vi "SLM Control.vi"(7 "Calling VI Ref":refnum<vi>) -> ()   [LabVIEW 2018]
uses:
  SLM Control TypeDefs/SLM Ctrl Mode Names.ctl
  <vilib>/Utility/miscctls.llb/LVPointTypeDef.ctl
  Device Library/Spatial Light Modulator/SLM Polymorphic Messenger/Get Status.vi
  Device Library/Spatial Light Modulator/SLM Polymorphic Messenger/Set Flat File.vi
  Device Library/Spatial Light Modulator/SLM Polymorphic Messenger/Number of Modes.vi
  Device Library/Spatial Light Modulator/SLM Polymorphic Messenger/Holo Size.vi
  Device Library/Spatial Light Modulator/SLM Polymorphic Messenger/Flat On or Off.vi
  Device Library/Spatial Light Modulator/SLM Polymorphic Messenger/Vortex On or Off.vi
  Device Library/Spatial Light Modulator/SLM Polymorphic Messenger/Toggle Vortex Direction.vi
  Device Library/Spatial Light Modulator/SLM Polymorphic Messenger/Top Hat On or Off.vi
  Device Library/Spatial Light Modulator/SLM Polymorphic Messenger/Top Hat Size.vi
  Device Library/Spatial Light Modulator/SLM Polymorphic Messenger/Mode Amplitude.vi
  Device Library/Spatial Light Modulator/SLM Polymorphic Messenger/Holo Position.vi
panel:
  out "Flat File":string
  in  "Center Holo":bool
  in  "X Pos Minus":bool
  in  "X Pos Plus":bool
  in  "Y Pos Minus":bool
  in  "Y Pos Plus":bool
  in  "Hologram Y Position":i32=20 min=1 max=1000
  in  "Hologram X Position":i32=20 min=1 max=1000
  in  "Set Flat File":bool
  in  "Clear All":bool
  in  "Set Zero":bool
  in  "Quit":bool
  in  "Notifier Name":string
  out "SLM Image":T1(plugin-control)
  in  "Active SLM":u16(ring) items=["Test"]
  in  "Hologram Diameter (px)":i32=20
  in  "Top Hat Radius":dbl=20.0
  in  "SLM Flat":bool
  in  "Vortex Direction":bool
  in  "Top Hap":bool
  in  "Mode Step Plus":bool
  in  "Mode Step Minus":bool
  in  "Current Mode":i32(ring) items=["Tip", "Tilt", "Defocus", "Astigmatism 90", "Astigmatism 45", "Coma 01", "Coma 02", "Trefoil 01", "Trefoil 02", "1st Spherical", "12", "13", "14", "15", "16", "17", "18", "19"]
  in  "Mode Amount":dbl
  in  "Step Size":dbl
  in  "Amp Step Plus":bool
  in  "Amp Step Minus":bool
  out "Error":bool
  in  "Number of Modes":i32=20 min=0 max=32
  in  "Vortex":bool
  out "Mode Plot":cluster{dbl[], dbl[]}(graph)
  # "SLM Display"
  # "Current Mode"
  # "Amplitude"
  # "Increment"
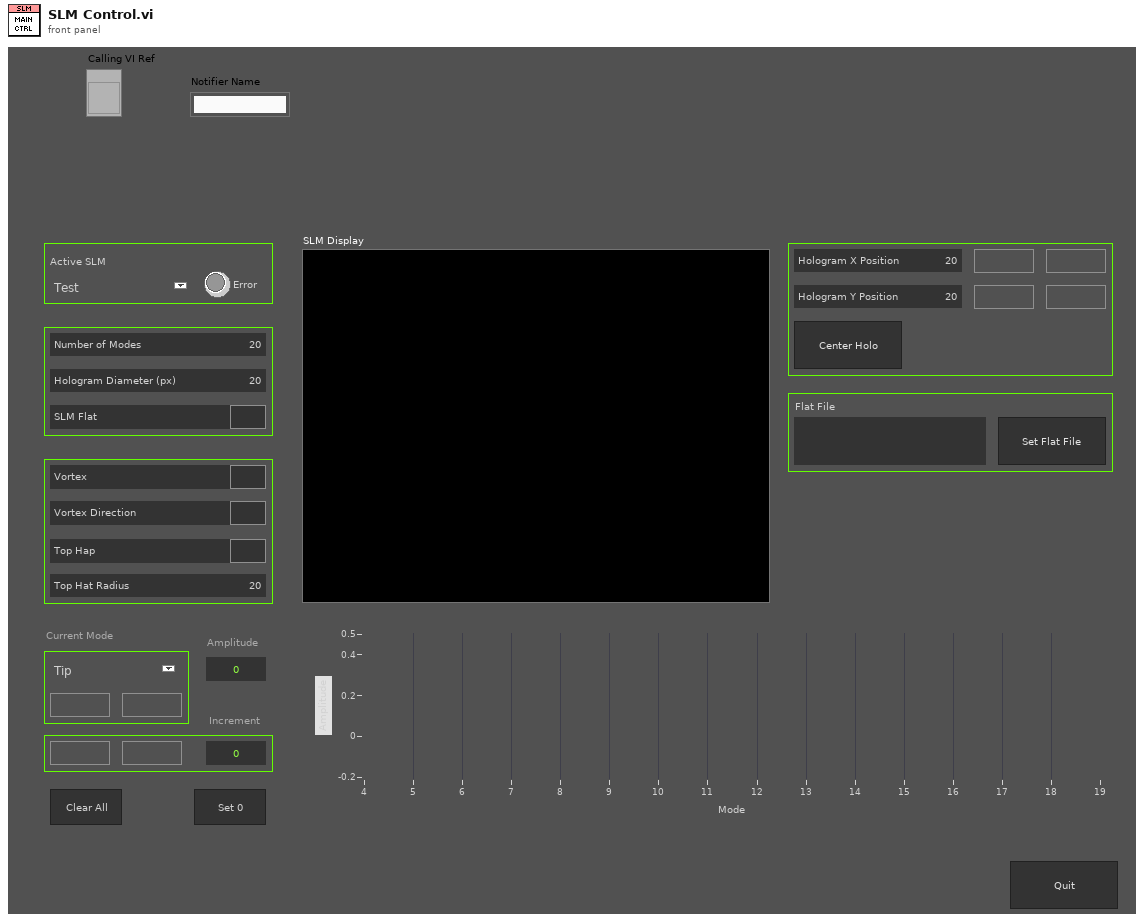
[diagram p1: front panel]
types:
  T1 = typedef "IMAQ Image.ctl" = refnum<image>
  T2 = enum16{"Always On", "Always Off", "Off While Running"}
  T3 = typedef "LVPointTypeDef.ctl" = cluster{"Horizontal":i16, "Vertical":i16}
  T4 = typedef "SLM Ctrl Mode Names.ctl" = cluster{"ModeNumbers":i32[], "ModeNames":string[]}
  T5 = typedef "X10468 SLM Notifier.ctl" = cluster{"SLM Actions":T6, "SLM Image":T1, "Flat On?":bool, "Vortex On?":bool, "Top Hat On?":bool, "Mode Amps":dbl[], "Number of Modes":i32, "Holo Diameter (px)":i32, "Top Hat Radius":dbl, "Holo Position":i32[], "Received?":bool, "Flat File Path":path}
  T6 = typedef "X10468 SLM Actions.ctl" = enum16{"Exit Loop", "Get Settings", "Set Flat File", "Change Holo Size", "Change Num Modes", "Change Holo Position", "Change Top Hat Size", "Change Vortex Direction", "Change Mode Amounts", "Flat On/Off", "Vortex On/Off", "Top Hat On/Off", "Make Hologram", "Update SLM Display", "Quit"}
  T7 = typedef "LVRectTypeDef.ctl" = cluster{"Left":i16, "Top":i16, "Right":i16, "Bottom":i16}
  T8 = typedef "LVBoundsTypeDef.ctl" = cluster{"Width":u32, "Height":u32}
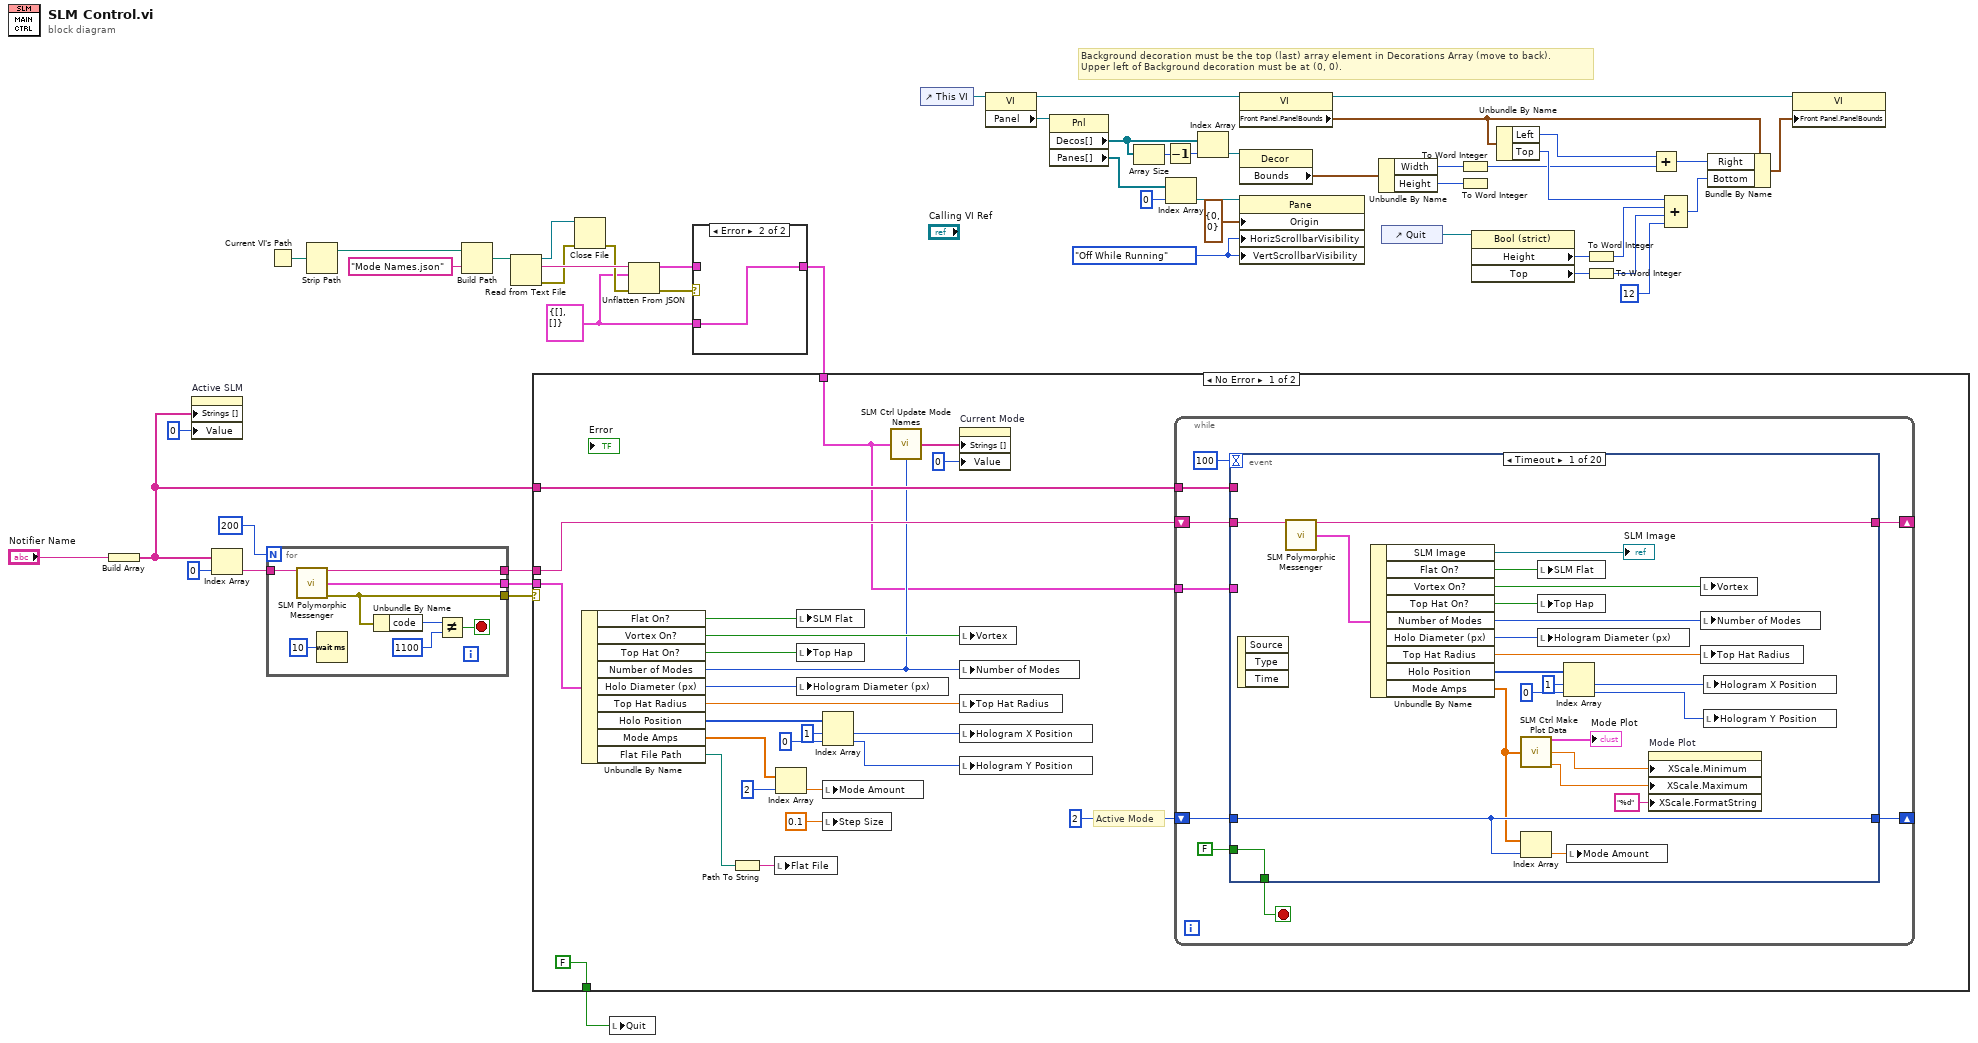
[diagram p0: block diagram]
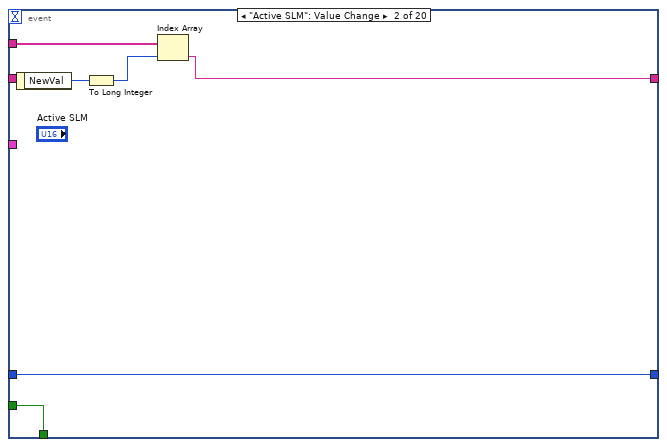
[diagram p2: hidden frame]
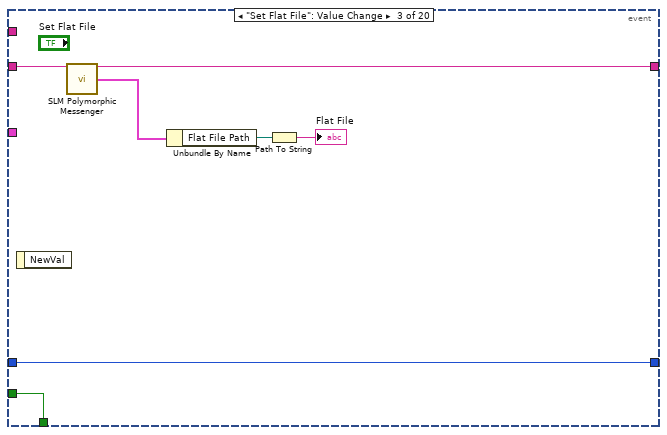
[diagram p3: hidden frame]
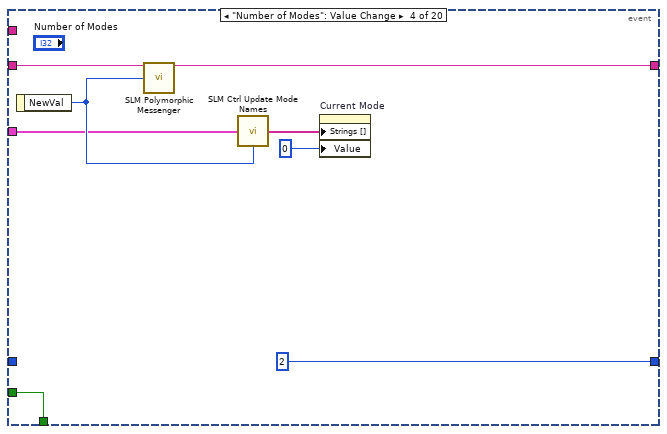
[diagram p4: hidden frame]
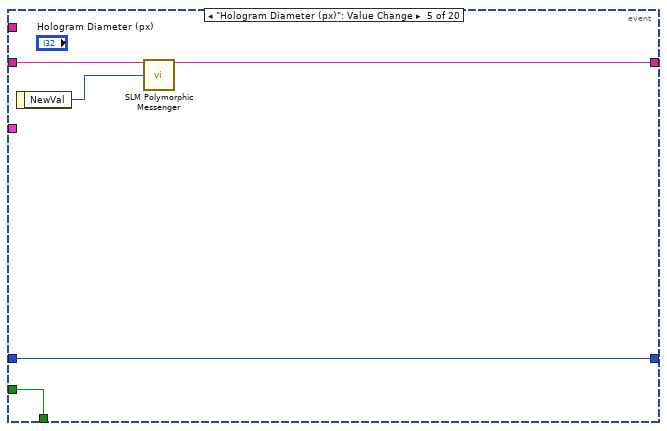
[diagram p5: hidden frame]
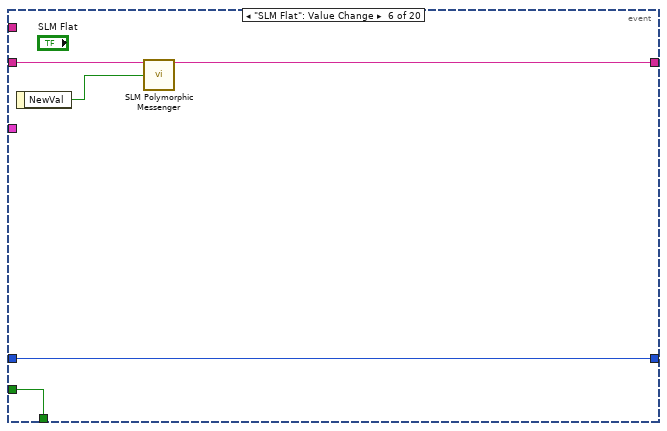
[diagram p6: hidden frame]
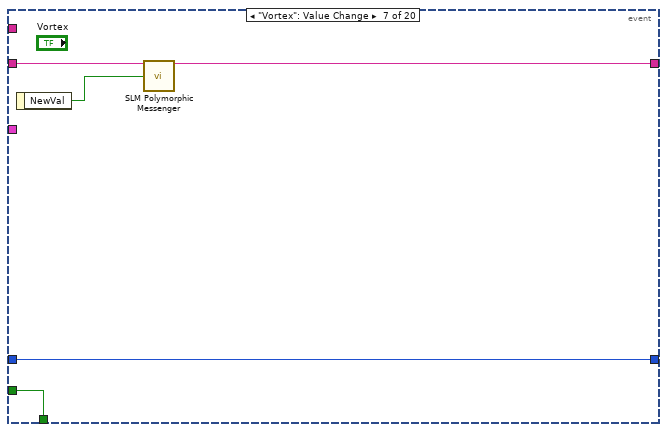
[diagram p7: hidden frame]
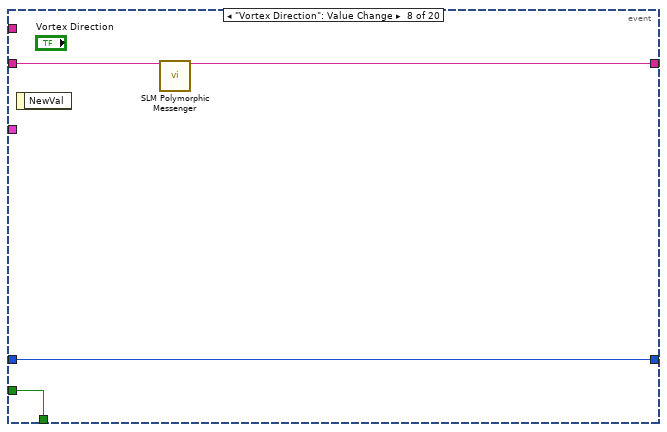
[diagram p8: hidden frame]
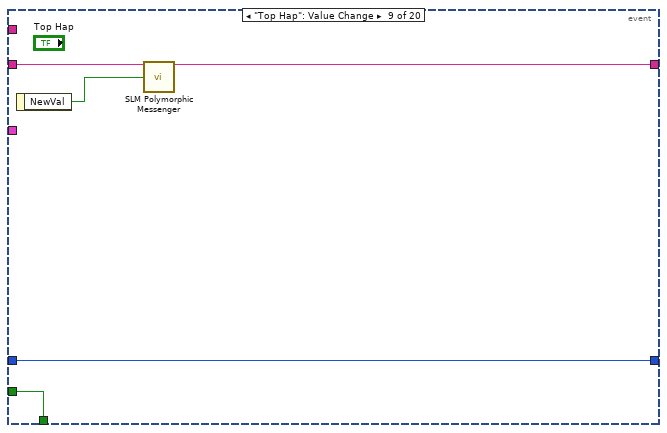
[diagram p9: hidden frame]
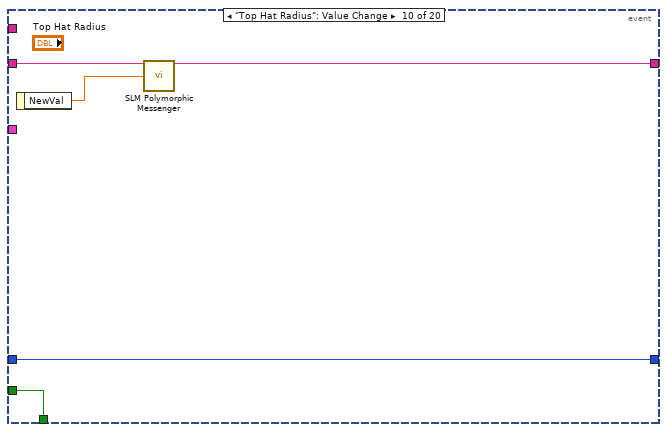
[diagram p10: hidden frame]
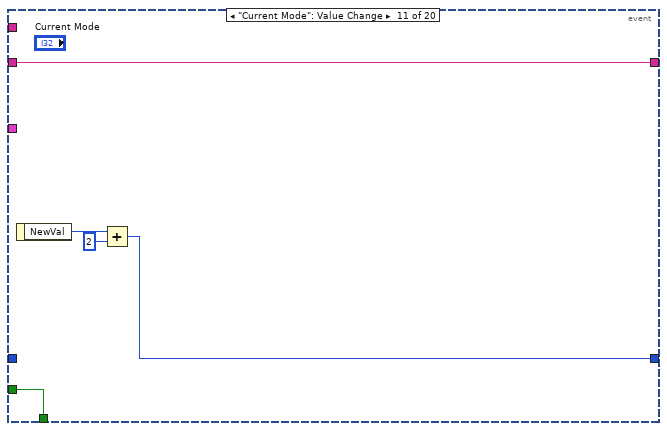
[diagram p11: hidden frame]
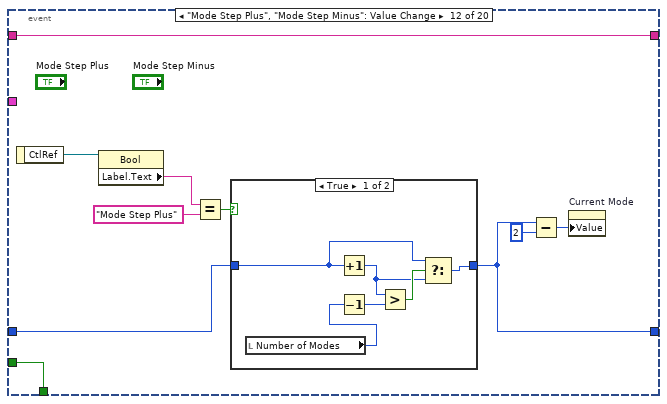
[diagram p12: hidden frame]
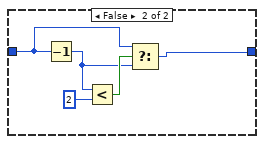
[diagram p13: hidden frame]
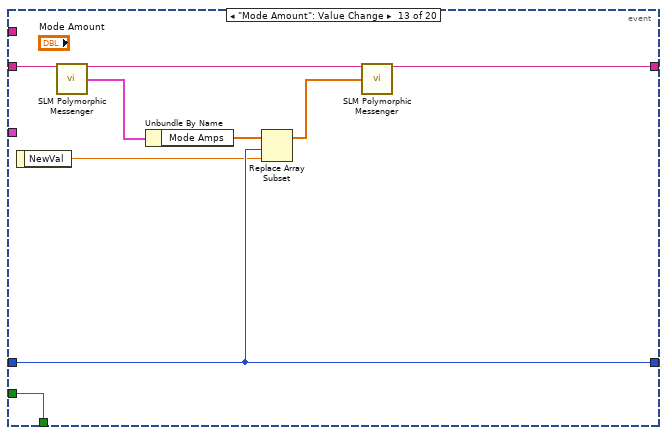
[diagram p14: hidden frame]
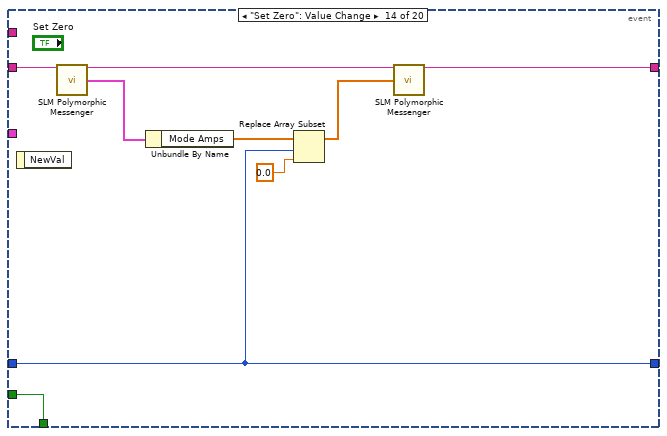
[diagram p15: hidden frame]
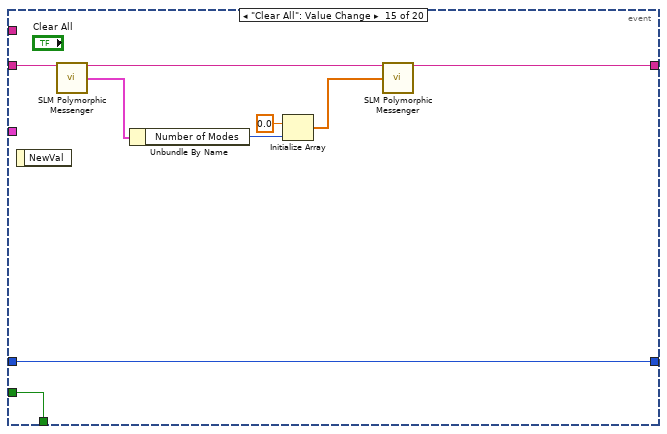
[diagram p16: hidden frame]
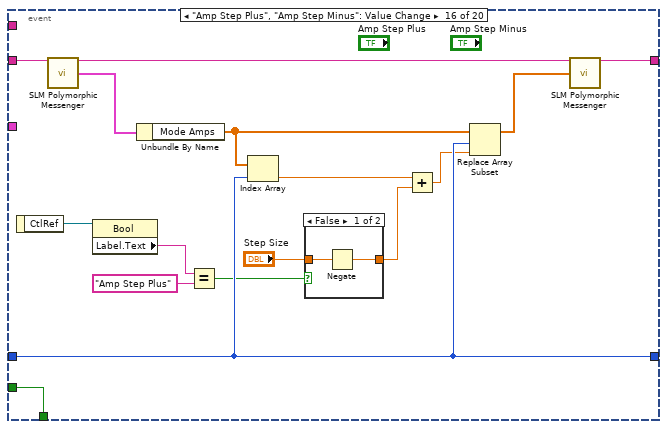
[diagram p17: hidden frame]
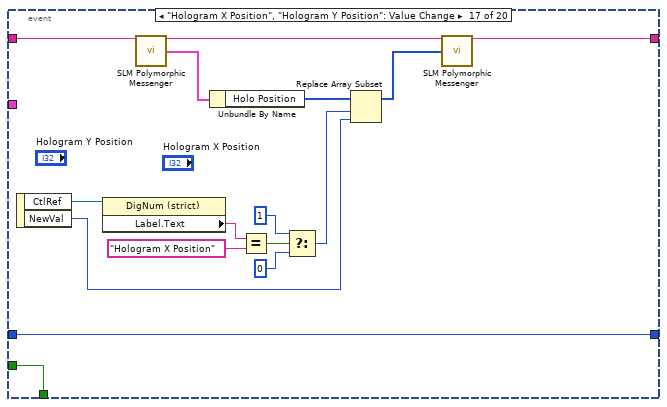
[diagram p19: hidden frame]
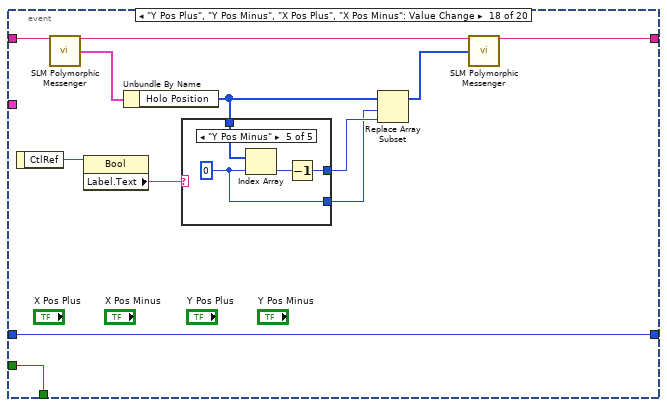
[diagram p20: hidden frame]
diagram:
  w12 = T2."Off While Running" ("Vertical Scrollbar Visibility")
  w37 = T4 {"ModeNumbers"=[], "ModeNames"=[]} ("ModeNamesArray")
  # "Background decoration must be the top (last) array element in Decorations Array (move to back).\nUpper left of Background decoration must be at (0, 0)."
  n1 = Build Array("Notifier Name") -> (w48:string[])
  n2 = property on="Active SLM" class="Ring (strict)"("Strings []"=w48, "Value"=u16 0) -> ()  [unwired: 2 in, 2 out]
  n3 = Index Array(array=w48, index=0) -> (element=w35:string)
  n4 = for {
    N: 200 -> [_]
    tunnel: [w56] -> w34
    tunnel: w35 -> [w54]
    tunnel: [w53] -> w33
    tunnel: [w52] -> w32
    stop <- w57 stop-if-true
    n5 = call-poly "SLM Polymorphic Messenger.vi"("Notifier Name"=w54) -> ("Notifier Name Dup"=w53:string, "SLM Status"=w52:T5, "Error Out"=w56:errorcluster)  [unwired: 12 in]
    n6 = Wait (ms)(milliseconds to wait=u32 10) -> ()  [unwired: 1 out]
    n7 = Unbundle By Name(w56) -> ("code"=w59:i32)
    n8 = Not Equal?(x=w59, y=1100 ("x")) -> (x != y?=w57:bool)
  }
  n9 = Current VI's Path() -> (path=w47:path)
  n10 = Strip Path(path=w47) -> (stripped path=w46:path)  [unwired: 1 out]
  n11 = Build Path(base path=w46, name or relative path="Mode Names.json") -> (appended path=w44:path)
  n12 = Read from Text File(file (use dialog)=w44) -> (refnum out=w42:refnum<file>, text=w43:string, error out=w41:errorcluster)  [unwired: 3 in, 1 out]
  n13 = Close File(refnum=w42, error in=w41) -> (error out=w40:errorcluster)  [unwired: 1 out]
  n14 = Unflatten From JSON(JSON string=w43, type and defaults=w37, error in (no error)=w40) -> (value=w38:T4, error out=w39:errorcluster)  [unwired: 4 in]
  n15 = case shown="Error" w39 {
    tunnel: w38 -> [w60 _]
    tunnel: [w60 w61] -> w31
    tunnel: w37 -> [_ w61]
    frame No Error {
    }
    frame Error {
    }
  }
  n16 = case shown="No Error" w34 {
    tunnel: w48 -> [w86 _]
    tunnel: w33 -> [w84 _]
    tunnel: w32 -> [w85 _]
    tunnel: w31 -> [w68 _]
    tunnel: [FALSE FALSE] -> w30
    frame No Error {
      # "Active Mode"
      n17 = Unbundle By Name(w85) -> ("Flat On?"=w83:bool, "Vortex On?"=w82:bool, "Top Hat On?"=w81:bool, "Number of Modes"=w72:i32, "Holo Diameter (px)"=w74:i32, "Top Hat Radius"=w73:dbl, "Holo Position"=w80:i32[], "Mode Amps"=w77:dbl[], "Flat File Path"=w63:path)
      n18 = Path To String(path=w63) -> (string=w62:string)
      n19 = local write "Flat File"(w62) -> ()
      n20 = Index Array(array=w77, index=2) -> (element=w75:dbl)
      n21 = local write "SLM Flat"(w83) -> ()
      n22 = local write "Top Hap"(w81) -> ()
      n23 = local write "Hologram Diameter (px)"(w74) -> ()
      n24 = Index Array(array=w80, index #1=1 ("index"), index #2=0 ("index")) -> (element #1=w65:i32, element #2=w66:i32)
      n25 = local write "Mode Amount"(w75) -> ()
      n26 = local write "Step Size"(0.1 ("Step Size")) -> ()
      n27 = call "SLM Ctrl Update Mode Names.vi"("ModeNamesArray"=w68, "Number of Modes"=w72) -> ("Mode Names"=w71:string[])  [unwired: 13 in]
      n28 = property on="Current Mode" class="Ring (strict)"("Strings []"=w71, "Value"=0 ("index")) -> ()  [unwired: 2 in, 2 out]
      n29 = local write "Vortex"(w82) -> ()
      n30 = local write "Number of Modes"(w72) -> ()
      n31 = local write "Top Hat Radius"(w73) -> ()
      n32 = local write "Hologram X Position"(w65) -> ()
      n33 = local write "Hologram Y Position"(w66) -> ()
      n34 = while {
        shift-right: [w91] -> _
        shift-left: w84 -> [w90]
        tunnel: w86 -> [w92]
        shift-right: [w89] -> _
        shift-left: 2 -> [w88]
        tunnel: w68 -> [w87]
        stop <- w93 stop-if-true
        n35 = event shown="[0] Timeout" {
          selector: _ -> [_ _ _ _ _ _ _ _ _ _ _ _ _ _ _ _ _ _ _ _]
          dyn-events: _ -> [_ _ _ _ _ _ _ _ _ _ _ _ _ _ _ _ _ _ _ _]
          timeout: 100 -> [_ _ _ _ _ _ _ _ _ _ _ _ _ _ _ _ _ _ _ _]
          tunnel: FALSE -> [w118 w124 w131 w139 w144 w149 w154 w158 w163 w168 w173 w183 w203 w212 w221 w237 w256 w268 w291 _]
          tunnel: [w118 w124 w131 w139 w144 w149 w154 w158 w163 w168 w173 w183 w203 w212 w221 w237 w256 w268 w291 TRUE] -> w93
          tunnel: w92 -> [_ w123 _ _ _ _ _ _ _ _ _ _ _ _ _ _ _ _ _ _]
          tunnel: [w116 w120 w128 w137 w142 w147 w152 w156 w161 w166 w172 w179 w196 w206 w216 w233 w253 w265 w290 w293] -> w91
          tunnel: w90 -> [w117 _ w129 w138 w143 w148 w153 w157 w162 w167 w172 w179 w202 w211 w220 w236 w255 w267 w288 w293]
          tunnel: [w104 w119 w130 2 ("index") w140 w145 w150 w155 w159 w164 w170 w176 w199 w208 w218 w227 w252 w264 w289 w292] -> w89
          tunnel: w88 -> [w104 w119 w130 _ w140 w145 w150 w155 w159 w164 _ w177 w199 w208 w218 w227 w252 w264 w289 w292]
          tunnel: w87 -> [_ _ _ w134 _ _ _ _ _ _ _ _ _ _ _ _ _ _ _ _]
          event Timeout {
            n36 = event-data() -> ()  [unwired: 1 in, 3 out]
            n37 = call-poly "SLM Polymorphic Messenger.vi"("Notifier Name"=w117) -> ("Notifier Name Dup"=w116:string, "SLM Status"=w105:T5)  [unwired: 12 in, 1 out]
            n38 = Unbundle By Name(w105) -> ("SLM Image"=→"SLM Image":T1, "Flat On?"=w106:bool, "Vortex On?"=w107:bool, "Top Hat On?"=w108:bool, "Number of Modes"=w115:i32, "Holo Diameter (px)"=w113:i32, "Top Hat Radius"=w114:dbl, "Holo Position"=w109:i32[], "Mode Amps"=w100:dbl[])
            n39 = call "SLM Ctrl Make Plot Data.vi"("Mode Array"=w100) -> ("Plot Data"=→"Mode Plot":cluster{dbl[], dbl[]}, "Min Value"=w98:dbl, "Max Value"=w97:dbl)  [unwired: 12 in]
            n40 = Index Array(array=w100, index=w104) -> (element=w112:dbl)
            n41 = local write "SLM Flat"(w106) -> ()
            n42 = local write "Top Hap"(w108) -> ()
            n43 = local write "Hologram Diameter (px)"(w113) -> ()
            n44 = Index Array(array=w109, index #1=1 ("index"), index #2=0 ("index")) -> (element #1=w102:i32, element #2=w101:i32)
            n45 = local write "Mode Amount"(w112) -> ()
            n46 = property on="Mode Plot" class="XYGraph (strict)"("XScale.Minimum"=w98, "XScale.Maximum"=w97, "XScale.FormatString"="%d" ("X Scale.Format String")) -> ()  [unwired: 2 in, 2 out]
            n47 = local write "Vortex"(w107) -> ()
            n48 = local write "Number of Modes"(w115) -> ()
            n49 = local write "Top Hat Radius"(w114) -> ()
            n50 = local write "Hologram X Position"(w102) -> ()
            n51 = local write "Hologram Y Position"(w101) -> ()
          }
          event "Active SLM": Value Change {
            n52 = event-data() -> ("NewVal"=w122:u16)  [unwired: 1 in]
            n53 = To Long Integer(number=w122) -> (32bit integer=w121:i32)
            n54 = Index Array(array=w123, index=w121) -> (element=w120:string)
          }
          event "Set Flat File": Value Change {
            n55 = event-data() -> ()  [unwired: 1 in, 1 out]
            n56 = call-poly "SLM Polymorphic Messenger.vi"("Notifier Name"=w129) -> ("Notifier Name Dup"=w128:string, "SLM Status"=w127:T5)  [unwired: 12 in, 1 out]
            n57 = Unbundle By Name(w127) -> ("Flat File Path"=w126:path)
            n58 = Path To String(path=w126) -> (string=→"Flat File":string)
          }
          event "Number of Modes": Value Change {
            n59 = event-data() -> ("NewVal"=w135:i32)  [unwired: 1 in]
            n60 = call-poly "SLM Polymorphic Messenger.vi"("Notifier Name"=w138, "Number of Modes"=w135) -> ("Notifier Name Dup"=w137:string)  [unwired: 11 in, 2 out]
            n61 = call "SLM Ctrl Update Mode Names.vi"("ModeNamesArray"=w134, "Number of Modes"=w135) -> ("Mode Names"=w136:string[])  [unwired: 13 in]
            n62 = property on="Current Mode" class="Ring (strict)"("Strings []"=w136, "Value"=0 ("index")) -> ()  [unwired: 2 in, 2 out]
          }
          event "Hologram Diameter (px)": Value Change {
            n63 = event-data() -> ("NewVal"=w141:i32)  [unwired: 1 in]
            n64 = call-poly "SLM Polymorphic Messenger.vi"("Notifier Name"=w143, "Holo Size (px)"=w141) -> ("Notifier Name Dup"=w142:string)  [unwired: 11 in, 2 out]
          }
          event "SLM Flat": Value Change {
            n65 = event-data() -> ("NewVal"=w146:bool)  [unwired: 1 in]
            n66 = call-poly "SLM Polymorphic Messenger.vi"("Notifier Name"=w148, "Flat On/Off"=w146) -> ("Notifier Name Dup"=w147:string)  [unwired: 11 in, 2 out]
          }
          event "Vortex": Value Change {
            n67 = event-data() -> ("NewVal"=w151:bool)  [unwired: 1 in]
            n68 = call-poly "SLM Polymorphic Messenger.vi"("Notifier Name"=w153, "Vortex On/Off"=w151) -> ("Notifier Name Dup"=w152:string)  [unwired: 11 in, 2 out]
          }
          event "Vortex Direction": Value Change {
            n69 = event-data() -> ()  [unwired: 1 in, 1 out]
            n70 = call-poly "SLM Polymorphic Messenger.vi"("Notifier Name"=w157) -> ("Notifier Name Dup"=w156:string)  [unwired: 12 in, 2 out]
          }
          event "Top Hap": Value Change {
            n71 = event-data() -> ("NewVal"=w160:bool)  [unwired: 1 in]
            n72 = call-poly "SLM Polymorphic Messenger.vi"("Notifier Name"=w162, "Top Hat On/Off"=w160) -> ("Notifier Name Dup"=w161:string)  [unwired: 11 in, 2 out]
          }
          event "Top Hat Radius": Value Change {
            n73 = event-data() -> ("NewVal"=w165:dbl)  [unwired: 1 in]
            n74 = call-poly "SLM Polymorphic Messenger.vi"("Notifier Name"=w167, "Top Hat Radius"=w165) -> ("Notifier Name Dup"=w166:string)  [unwired: 11 in, 2 out]
          }
          event "Current Mode": Value Change {
            n75 = event-data() -> ("NewVal"=w171:i32)  [unwired: 1 in]
            n76 = Add(x=w171, y=2) -> (x+y=w170:i32)
          }
          event "Mode Step Plus", "Mode Step Minus": Value Change {
            n77 = event-data() -> ("CtlRef"=w182:refnum<vi>)  [unwired: 1 in]
            n78 = property class="Bool"(reference=w182) -> ("Label.Text"=w181:string)  [unwired: 1 in, 2 out]
            n79 = Equal?(x=w181, y="Mode Step Plus") -> (x = y?=w178:bool)
            n80 = case shown="True" w178 {
              tunnel: w177 -> [w188 w193]
              tunnel: [w186 w191] -> w176
              frame True {
                n81 = local read "Number of Modes"() -> (w184:i32)
                n82 = Increment(x=w188) -> (x+1=w187:i32)
                n83 = Decrement(x=w184) -> (x-1=w185:i32)
                n84 = Greater?(x=w187, y=w185) -> (0:w189:bool)
                n85 = Select(t=w188, s=w189, f=w187) -> (s? t:f=w186:i32)
              }
              frame False {
                n86 = Decrement(x=w193) -> (x-1=w192:i32)
                n87 = Less?(x=w192, y=2) -> (x < y?=w194:bool)
                n88 = Select(t=w193, s=w194, f=w192) -> (s? t:f=w191:i32)
              }
            }
            n89 = Subtract(x=w176, y=2) -> (x-y=w175:i32)
            n90 = property on="Current Mode" class="Ring (strict)"("Value"=w175) -> ()  [unwired: 2 in, 2 out]
          }
          event "Mode Amount": Value Change {
            n91 = event-data() -> ("NewVal"=w198:dbl)  [unwired: 1 in]
            n92 = call-poly "SLM Polymorphic Messenger.vi"("Notifier Name"=w202) -> ("Notifier Name Dup"=w197:string, "SLM Status"=w201:T5)  [unwired: 12 in, 1 out]
            n93 = Unbundle By Name(w201) -> ("Mode Amps"=w200:dbl[])
            n94 = Replace Array Subset(array=w200, new element=w198, index=w199) -> (w195:dbl[])
            n95 = call-poly "SLM Polymorphic Messenger.vi"("Notifier Name"=w197, "Mode Amounts"=w195) -> ("Notifier Name Dup"=w196:string)  [unwired: 11 in, 2 out]
          }
          event "Set Zero": Value Change {
            n96 = event-data() -> ()  [unwired: 1 in, 1 out]
            n97 = call-poly "SLM Polymorphic Messenger.vi"("Notifier Name"=w211) -> ("Notifier Name Dup"=w207:string, "SLM Status"=w210:T5)  [unwired: 12 in, 1 out]
            n98 = Unbundle By Name(w210) -> ("Mode Amps"=w209:dbl[])
            n99 = Replace Array Subset(array=w209, new element=0.0 ("new element/subarray"), index=w208) -> (w205:dbl[])
            n100 = call-poly "SLM Polymorphic Messenger.vi"("Notifier Name"=w207, "Mode Amounts"=w205) -> ("Notifier Name Dup"=w206:string)  [unwired: 11 in, 2 out]
          }
          event "Clear All": Value Change {
            n101 = event-data() -> ()  [unwired: 1 in, 1 out]
            n102 = call-poly "SLM Polymorphic Messenger.vi"("Notifier Name"=w220) -> ("Notifier Name Dup"=w217:string, "SLM Status"=w219:T5)  [unwired: 12 in, 1 out]
            n103 = Unbundle By Name(w219) -> ("Number of Modes"=w215:i32)
            n104 = Initialize Array(0.0 ("element"), w215) -> (w213:dbl[])
            n105 = call-poly "SLM Polymorphic Messenger.vi"("Notifier Name"=w217, "Mode Amounts"=w213) -> ("Notifier Name Dup"=w216:string)  [unwired: 11 in, 2 out]
          }
          event "Amp Step Plus", "Amp Step Minus": Value Change {
            n106 = event-data() -> ("CtlRef"=w229:refnum<vi>)  [unwired: 1 in]
            n107 = call-poly "SLM Polymorphic Messenger.vi"("Notifier Name"=w236) -> ("Notifier Name Dup"=w234:string, "SLM Status"=w235:T5)  [unwired: 12 in, 1 out]
            n108 = property class="Bool"(reference=w229) -> ("Label.Text"=w231:string)  [unwired: 1 in, 2 out]
            n109 = Unbundle By Name(w235) -> ("Mode Amps"=w228:dbl[])
            n110 = Equal?(x=w231, y="Amp Step Plus") -> (x = y?=w224:bool)
            n111 = Index Array(array=w228, index=w227) -> (element=w226:dbl)
            n112 = case shown="False" w224 {
              tunnel: "Step Size" -> [w239 w240]
              tunnel: [w238 w240] -> w222
              frame False {
                n113 = Negate(x=w239) -> (-x=w238:dbl)
              }
              frame True {
              }
            }
            n114 = Add(x=w226, y=w222) -> (x+y=w225:dbl)
            n115 = Replace Array Subset(array=w228, new element=w225, index=w227) -> (w232:dbl[])
            n116 = call-poly "SLM Polymorphic Messenger.vi"("Notifier Name"=w234, "Mode Amounts"=w232) -> ("Notifier Name Dup"=w233:string)  [unwired: 11 in, 2 out]
          }
          event "Hologram X Position", "Hologram Y Position": Value Change {
            n117 = event-data() -> ("CtlRef"=w250:refnum<vi>, "NewVal"=w245:i32)  [unwired: 1 in]
            n118 = property class="DigNum (strict)"(reference=w250) -> ("Label.Text"=w249:string)  [unwired: 1 in, 2 out]
            n119 = call-poly "SLM Polymorphic Messenger.vi"("Notifier Name"=w255) -> ("Notifier Name Dup"=w254:string, "SLM Status"=w251:T5)  [unwired: 12 in, 1 out]
            n120 = Unbundle By Name(w251) -> ("Holo Position"=w247:i32[])
            n121 = Equal?(x=w249, y="Hologram X Position") -> (x = y?=w244:bool)
            n122 = Select(t=1, s=w244, f=0) -> (s? t:f=w241:i32)
            n123 = Replace Array Subset(array=w247, new element=w245, index=w241) -> (w246:i32[])
            n124 = call-poly "SLM Polymorphic Messenger.vi"("Notifier Name"=w254, "Holo Position"=w246) -> ("Notifier Name Dup"=w253:string)  [unwired: 11 in, 2 out]
          }
          event "Y Pos Plus", "Y Pos Minus", "X Pos Plus", "X Pos Minus": Value Change {
            n125 = event-data() -> ("CtlRef"=w262:refnum<vi>)  [unwired: 1 in]
            n126 = call-poly "SLM Polymorphic Messenger.vi"("Notifier Name"=w267) -> ("Notifier Name Dup"=w266:string, "SLM Status"=w263:T5)  [unwired: 12 in, 1 out]
            n127 = property class="Bool"(reference=w262) -> ("Label.Text"=w260:string)  [unwired: 1 in, 2 out]
            n128 = Unbundle By Name(w263) -> ("Holo Position"=w258:i32[])
            n129 = case shown="\"Y Pos Minus\"" w260 {
              tunnel: [0 w274 w278 w282 w286] -> w259
              tunnel: w258 -> [_ w273 w277 w281 w285]
              tunnel: [0 ("index") w271 w275 w279 w283] -> w257
              frame Default {
              }
              frame "X Pos Plus" {
                w271 = 1 ("index")
                n130 = Index Array(array=w273, index=w271) -> (element=w272:i32)
                n131 = Increment(x=w272) -> (x+1=w274:i32)
              }
              frame "X Pos Minus" {
                w275 = 1 ("index")
                n132 = Index Array(array=w277, index=w275) -> (element=w276:i32)
                n133 = Decrement(x=w276) -> (x-1=w278:i32)
              }
              frame "Y Pos Plus" {
                w279 = 0 ("index")
                n134 = Index Array(array=w281, index=w279) -> (element=w280:i32)
                n135 = Increment(x=w280) -> (x+1=w282:i32)
              }
              frame "Y Pos Minus" {
                w283 = 0 ("index")
                n136 = Index Array(array=w285, index=w283) -> (element=w284:i32)
                n137 = Decrement(x=w284) -> (x-1=w286:i32)
              }
            }
            n138 = Replace Array Subset(array=w258, new element=w259, index=w257) -> (w261:i32[])
            n139 = call-poly "SLM Polymorphic Messenger.vi"("Notifier Name"=w266, "Holo Position"=w261) -> ("Notifier Name Dup"=w265:string)  [unwired: 11 in, 2 out]
          }
          event "Center Holo": Value Change {
            n140 = event-data() -> ()  [unwired: 1 in, 1 out]
            n141 = call-poly "SLM Polymorphic Messenger.vi"("Notifier Name"=w288, "Holo Position"=i32[] [300, 396]) -> ("Notifier Name Dup"=w290:string)  [unwired: 11 in, 2 out]
          }
          event "Quit": Value Change {
            n142 = event-data() -> ()  [unwired: 1 in, 1 out]
          }
        }
      }
    }
    frame Error {
    }
  }
  n143 = local write "Quit"(w30) -> ()
  n144 = control-ref of="This VI"() -> (w4:refnum<vi>)
  n145 = property class="VI"(reference=w4) -> (reference out=w13:refnum<vi>, "Panel"=w5:refnum<vi>)  [unwired: 1 in, 1 out]
  n146 = property class="Pnl"(reference=w5) -> ("Decos[]"=w3:refnum<vi>[], "Panes[]"=w9:refnum<vi>[])  [unwired: 1 in, 2 out]
  n147 = Array Size(array=w3) -> (size(s)=w1:i32)
  n148 = Decrement(x=w1) -> (x-1=w2:i32)
  n149 = Index Array(array=w9, index=0) -> (element=w8:refnum<vi>)
  n150 = Index Array(array=w3, index=w2) -> (element=w11:refnum<vi>)
  n151 = property class="VI"(reference=w13) -> (reference out=w15:refnum<vi>, "Front Panel.PanelBounds"=w16:T7)  [unwired: 1 in, 1 out]
  n152 = property class="Decor"(reference=w11) -> ("Bounds"=w14:T8)  [unwired: 1 in, 2 out]
  n153 = property class="Pane"(reference=w8, "Origin"=T3 {"Horizontal"=0, "Vertical"=0}, "HorizScrollbarVisibility"=w12, "VertScrollbarVisibility"=w12) -> ()  [unwired: 1 in, 2 out]
  n154 = Unbundle By Name(w14) -> ("Width"=w19:u32, "Height"=w22:u32)
  n155 = control-ref of="Quit"() -> (w6:refnum<vi>)
  n156 = To Word Integer(number=w19) -> (16bit integer=w21:i16)
  n157 = To Word Integer(number=w22) -> ()  [unwired: 1 out]
  n158 = property class="Bool (strict)"(reference=w6) -> ("Height"=w24:u32, "Top"=w25:i32)  [unwired: 1 in, 2 out]
  n159 = Unbundle By Name(w16) -> ("Left"=w18:i16, "Top"=w29:i16)
  n160 = To Word Integer(number=w24) -> (16bit integer=w27:i16)
  n161 = To Word Integer(number=w25) -> (16bit integer=w28:i16)
  n162 = Add(x=w18, y=w21) -> (x+y=w20:i16)
  n163 = Compound Arithmetic op=ADD(w29, w27, w28, i16 12 ("y")) -> (w23:i16)
  n164 = Bundle By Name(cluster=w16, "Right"=w20, "Bottom"=w23) -> (w17:T7)
  n165 = property class="VI"(reference=w15, "Front Panel.PanelBounds"=w17) -> ()  [unwired: 1 in, 2 out]
